vi "ConnectionHandler.vi"(11 "connection ID":refnum<k5>) -> ()   [LabVIEW 2013, in "WebSockets.lvlib"]
uses:
  WebSockets.lvlib
  ConnectionHandlerStates.ctl
  ReadMessage.ctl
panel:
  in  "user event in":refnum<user-event>
  out "Data":string
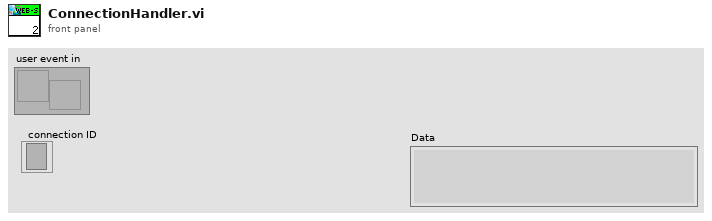
[diagram p1: front panel]
types:
  T1 = typedef "WebSockets.lvlib/ConnectionHandlerStates.ctl" = enum16{"Handshake", "Listening", "Exit"}
  T2 = typedef "WebSockets.lvlib/ReadMessage.ctl" = cluster{"ConnectionID":string, "Data":string}
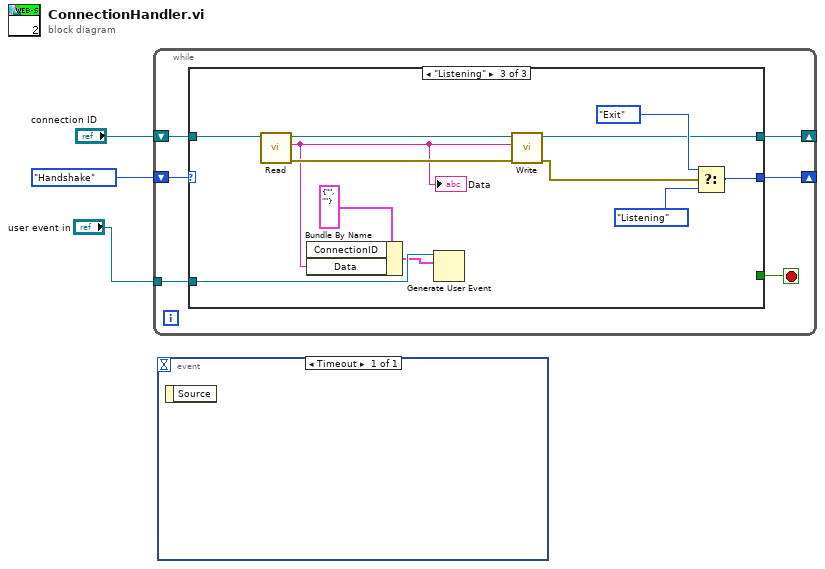
[diagram p0: block diagram]
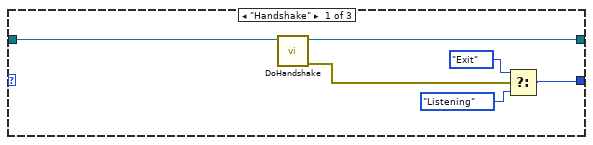
[diagram p2: hidden frame]
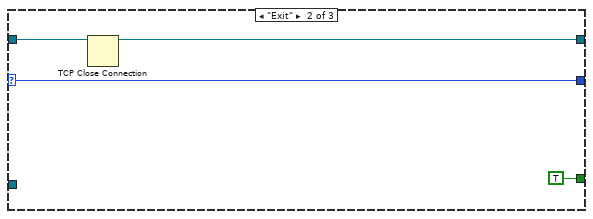
[diagram p3: hidden frame]
diagram:
  n1 = while {
    shift-right: [w5] -> _
    shift-left: "connection ID" -> [w9]
    shift-right: [w7] -> _
    shift-left: ConnectionHandlerStates."Handshake" -> [w8]
    tunnel: "user event in" -> [w4]
    stop <- w6 stop-if-true
    n2 = case shown="\"Listening\"" w8 {
      selector: w8 -> [_ w18 _]
      tunnel: w9 -> [w15 w17 w31]
      tunnel: [w11 w18 w30] -> w7
      tunnel: [_ TRUE _] -> w6
      tunnel: [w14 w16 w26] -> w5
      tunnel: w4 -> [_ _ w22]
      frame "Handshake" {
        n3 = call "DoHandshake.vi"("TCP Network Connection in"=w15) -> ("error out"=w10:errorcluster, "TCP Network Connection out"=w14:refnum<k5>)  [unwired: 8 in, 1 out]
        n4 = Select(t=ConnectionHandlerStates."Exit", s=w10, f=ConnectionHandlerStates."Listening") -> (s? t:f=w11:T1)
      }
      frame "Exit" {
        n5 = TCP Close Connection(connection ID=w17) -> (connection ID out=w16:refnum<k5>)  [unwired: 2 in, 1 out]
      }
      frame "Listening" {
        n6 = call "Read.vi"("connection ID"=w31) -> ("error out"=w25:errorcluster, "Data"=w21:string, "connection ID out"=w27:refnum<k5>)  [unwired: 7 in, 1 out]
        "Data" <- w21
        n7 = Bundle By Name(cluster=T2 {"ConnectionID"="", "Data"=""}, "Data"=w21) -> (w20:T2)  [unwired: 1 in]
        n8 = Generate User Event(user event=w22, event data cluster=w20) -> ()  [unwired: 2 in, 2 out]
        n9 = call "Write.vi"("error in (no error)"=w25, "Data"=w21, "connection ID"=w27) -> ("error out"=w24:errorcluster, "connection ID out"=w26:refnum<k5>)  [unwired: 7 in]
        n10 = Select(t=ConnectionHandlerStates."Exit", s=w24, f=ConnectionHandlerStates."Listening") -> (s? t:f=w30:T1)
      }
    }
  }
  n11 = event shown="[0] Timeout" {
    selector: _ -> [_]
    dyn-events: _ -> [_]
    timeout: _ -> [_]
    event Timeout {
      n12 = event-data() -> ()  [unwired: 1 in, 1 out]
    }
  }
